vi "PicohrdlUnitInfo.vi"(8 "error in (no error)":errorcluster, 11 "handle in":i16) -> (0 "error out":errorcluster, 2 "Unit Info":T1, 3 "handle out":i16)   [LabVIEW 2010]
doc: "Calls HRDLGetUnitInfo() in a loop to all unit Info from device."
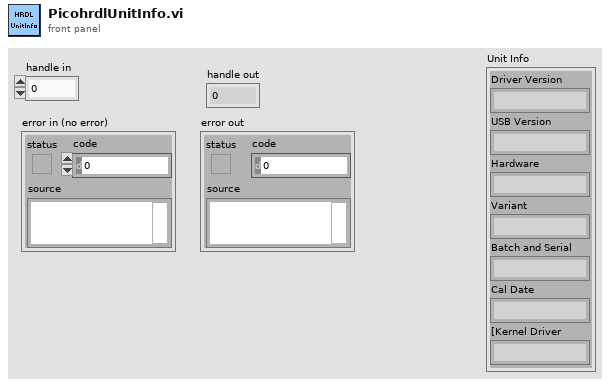
[diagram p1: front panel]
types:
  T1 = cluster{"Driver Version":string, "USB Version":string, "Hardware":string, "Variant":string, "Batch and Serial":string, "Cal Date":string, "[Kernel Driver":string, "[7]":string, "[8]":string, "[9]":string, "[10]":string, "[11]":string, "[12]":string, "[13]":string, "[14]":string}
  T2 = cluster{"[0]":string, "[1]":string, "[2]":string, "[3]":string, "[4]":string, "[5]":string, "[6]":string, "[7]":string, "[8]":string, "[9]":string, "[10]":string, "[11]":string, "[12]":string, "[13]":string, "[14]":string}
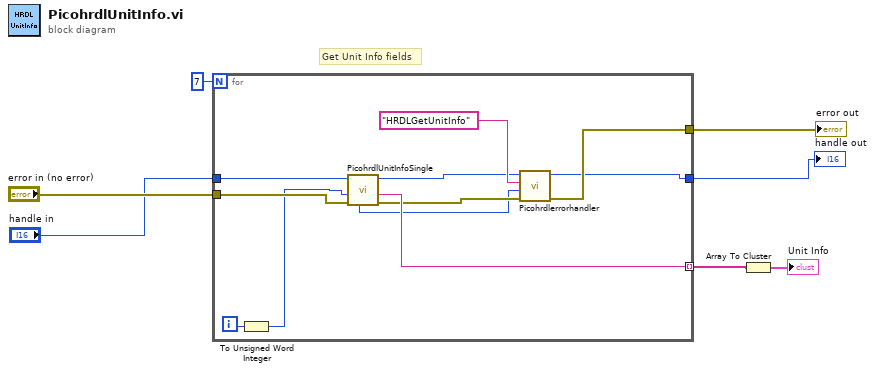
[diagram p0: block diagram]
diagram:
  # "Get Unit Info fields"
  n1 = for {
    N: 7 -> [_]
    tunnel: "error in (no error)" -> [w18]
    tunnel: "handle in" -> [w17]
    tunnel: [w16] -> w4 mode=indexing
    tunnel: [w10] -> w3
    tunnel: [w11] -> w2
    i -> [w15]
    n2 = To Unsigned Word Integer(number=w15) -> (unsigned 16bit integer=w14:u16)
    n3 = call "PicohrdlUnitInfoSingle.vi"("error in (no error)"=w18, "info Enum"=w14, "Handle in"=w17) -> ("error out"=w12:errorcluster, "trimmed string"=w16:string, "handle out"=w9:i16, "status"=w8:i16)  [unwired: 5 in]
    n4 = call "Picohrdlerrorhandler.vi"("Handle in"=w9, "API function"="HRDLGetUnitInfo", "Return"=w8, "error in (no error)"=w12) -> ("Handle out"=w10:i16, "error out"=w11:errorcluster)  [unwired: 5 in]
  }
  "error out" <- w2
  "handle out" <- w3
  n5 = Array To Cluster(array=w4) -> (cluster=→"Unit Info":T2)
